vi "Utility Create Binary String.vi"(10 "Input Array":i16[](array[numeric])) -> (2 "Binary String":string)   [LabVIEW 2012, in "Agilent ESG Series.lvlib"]
doc: "This VI convert binary data array to binary VISA string for transfer into instrument.\n\nOutput Binary string:\n\n#ABC\n\nA the number of decimal digits to follow in B.\nB a decimal number specifying the number of data bytes in C.\nC the binary waveform data."
uses:
  <instrlib>/Agilent ESG Series/Agilent ESG Series.lvlib
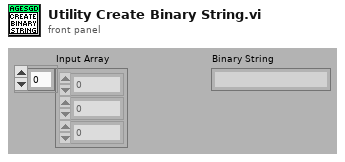
[diagram p1: front panel]
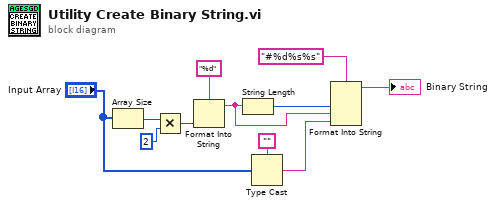
[diagram p0: block diagram]
diagram:
  n1 = Array Size(array="Input Array") -> (size(s)=w11:i32)
  n2 = Multiply(x=w11, y=2) -> (x*y=w9:i32)
  n3 = Format Into String(format string="%d", w9) -> (resulting string=w6:string)  [unwired: 2 in, 1 out]
  n4 = String Length(string=w6) -> (length=w7:i32)
  n5 = Type Cast(type="", x="Input Array") -> (*(type *) &x=w3:string)
  n6 = Format Into String(format string="#%d%s%s", w7, w6, w3) -> (resulting string=→"Binary String":string)  [unwired: 2 in, 1 out]
